vi "Stop Core.vi"(10 "final error code":i32, 11 "Waveform_Task in":refnum<class "Waveform_Task.lvclass">) -> (3 "Waveform_Task out":refnum<class "Waveform_Task.lvclass">)   [LabVIEW 2025, in "Waveform_Task.lvlib" / "Waveform_Task.lvclass"]
doc: "<p>(<strong>Filename</strong>: <span class=\"dnl\">Actor Framework.lvlib:Actor.lvclass:Stop Core.vi</span>)</p>\n<p>Defines what the actor does before it stops. Use the <strong>final error code</strong> input to determine whether the actor shut down in response to an error.</p>\n<p>By default, this method passes the Stop message along to all <a href=\"nihelplauncher://docs/csh?context=lvcore_lvcomm_af_launch_nested_actor\">auto-stop nested actors</a>. A descendant class may override this method to define additional behavior, such as shutting down any processes the actor initiated in its override of the <a href=\"nihelplauncher://docs/csh?context=lvcore_lvcomm_af_actor_core\">Actor Core</a> method.</p>"
uses:
  Waveform_Task.lvclass
  Waveform_Task.lvclass/Waveform_Task.ctl
  Task_Abstr/Task_Abstr/Task_Abstr.lvclass
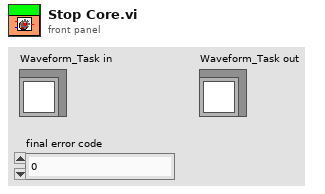
[diagram p1: front panel]
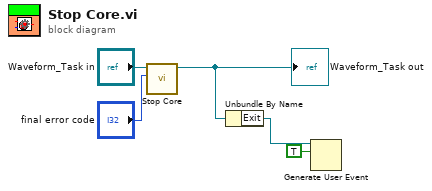
[diagram p0: block diagram]
diagram:
  n1 = call-parent "Stop Core.vi"("final error code"="final error code", "Task_Abstr in"="Waveform_Task in") -> ("Task_Abstr out"=w2:refnum<class "Waveform_Task.lvclass">)  [unwired: 9 in]
  "Waveform_Task out" <- w2
  n2 = Unbundle By Name(w2) -> ("Exit"=w1:refnum<user-event>)
  n3 = Generate User Event(user event=w1, event data cluster=TRUE ("event data")) -> ()  [unwired: 2 in, 2 out]
